vi "释放所有通道.vi"(9 "RF/CLK":string, 11 "TCP Network Connection in":refnum<k5>) -> (0 "error out":errorcluster, 3 "TCP Network Connection out":refnum<k5>)   [LabVIEW 2015]
uses:
  Global/SeverGlobal.vi
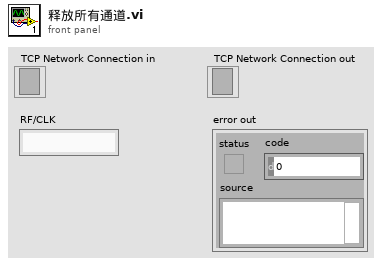
[diagram p1: front panel]
types:
  T1 = typedef "响应消息头.ctl" = string
  T2 = cluster{"TCP Ref":refnum<k5>, "IP":string, "userName":string, "A":u16, "COM":u16, "time":u32}[]
  T3 = cluster{"TCP Ref":refnum<k5>, "Broadcast":refnum<k5>, "TF Ref":refnum<k5>, "IP":string, "port":u16, "userName":string, "passWord":string, "authority":string}[]
  T4 = cluster{"TCP Ref":refnum<k5>, "IP":string, "userName":string, "IN":u16, "OUT":u16, "time":u32}[]
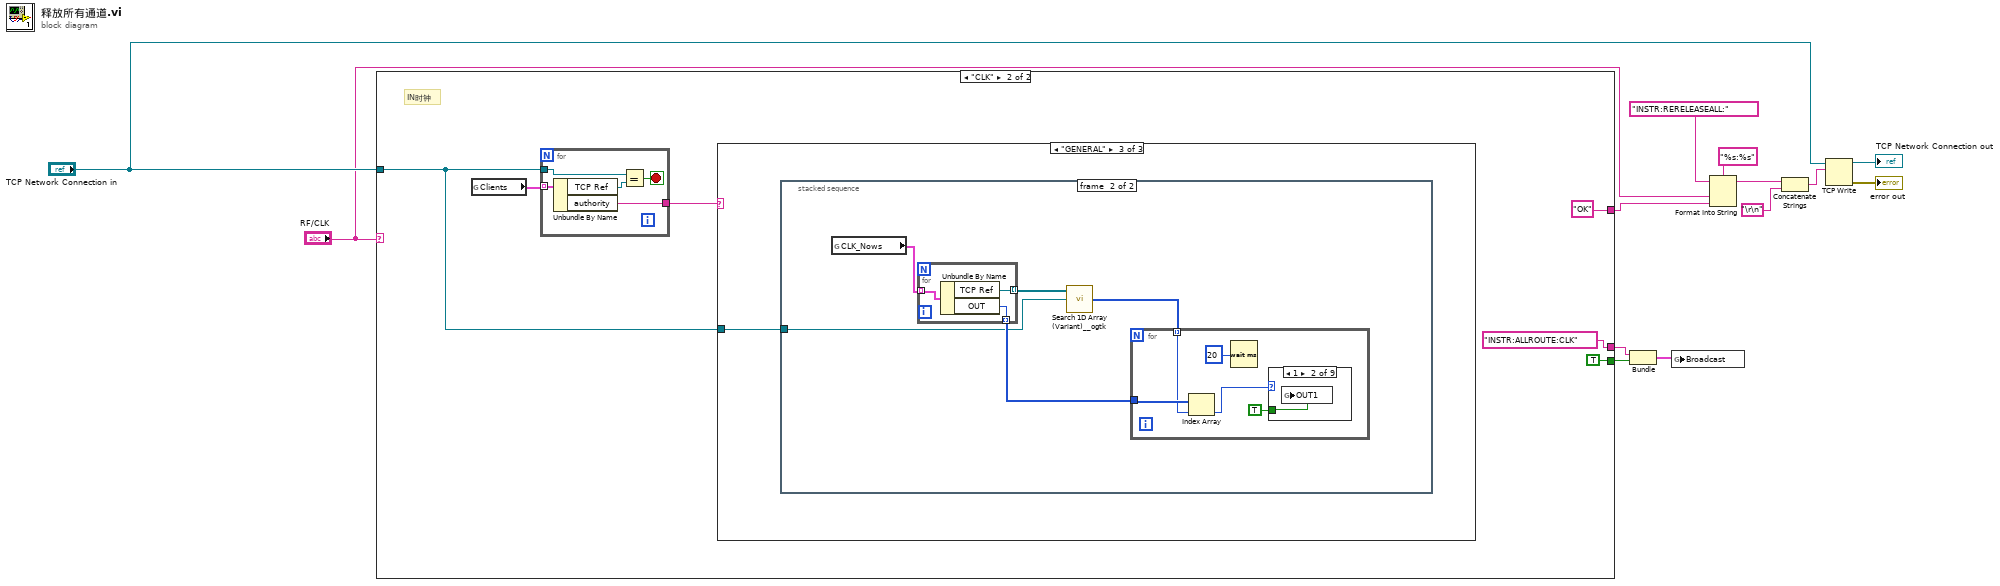
[diagram p0: block diagram]
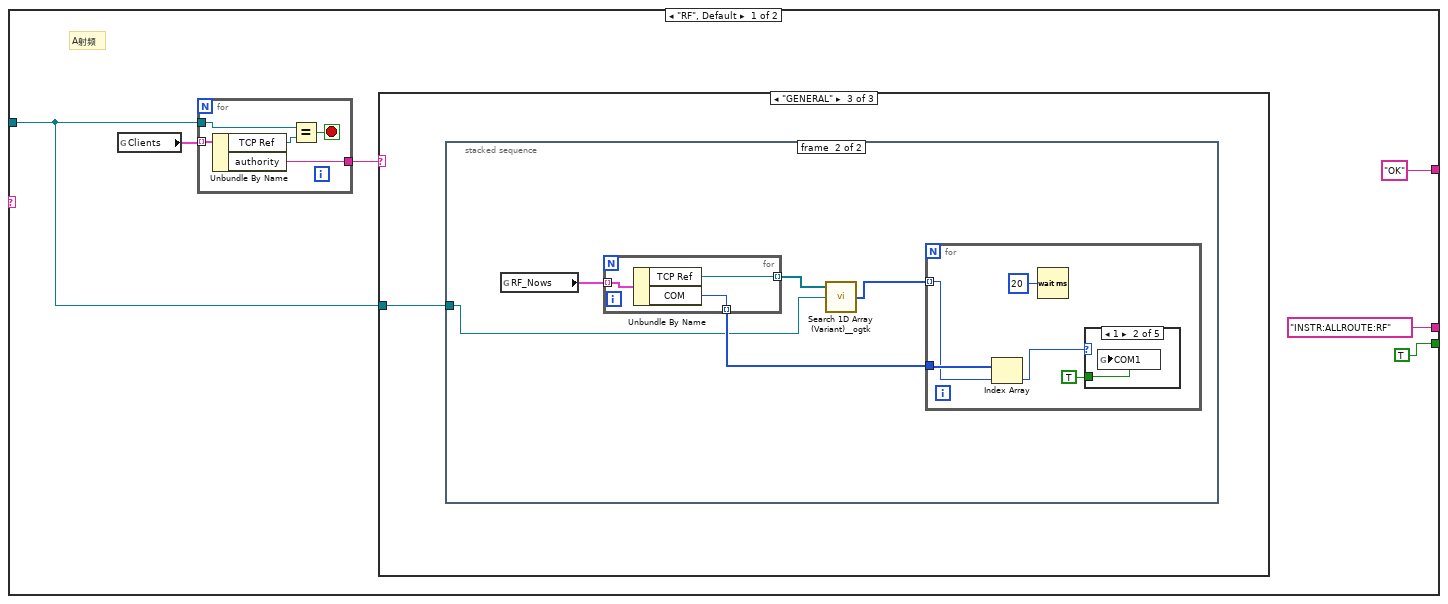
[diagram p2: hidden frame]
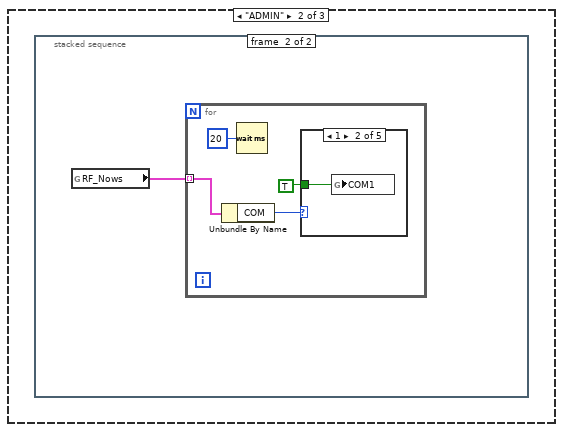
[diagram p4: hidden frame]
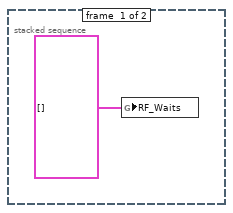
[diagram p5: hidden frame]
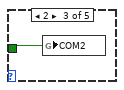
[diagram p7: hidden frame]
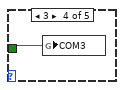
[diagram p8: hidden frame]
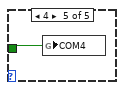
[diagram p9: hidden frame]
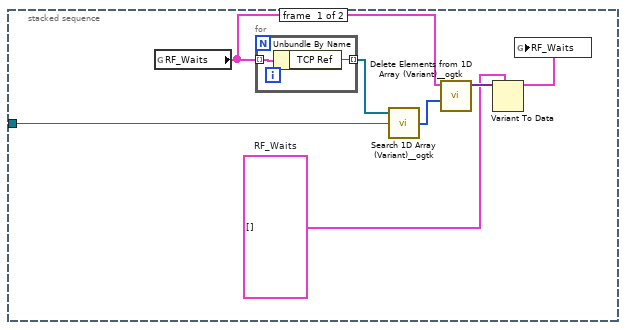
[diagram p10: hidden frame]
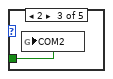
[diagram p12: hidden frame]
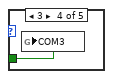
[diagram p13: hidden frame]
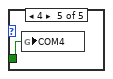
[diagram p14: hidden frame]
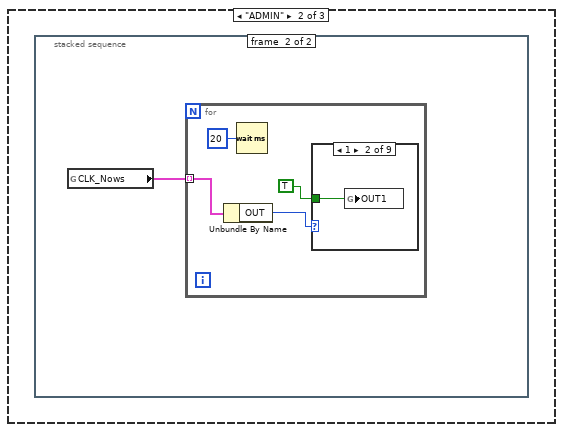
[diagram p16: hidden frame]
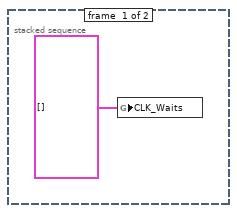
[diagram p17: hidden frame]
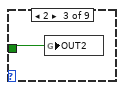
[diagram p19: hidden frame]
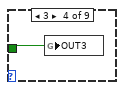
[diagram p20: hidden frame]
diagram:
  n1 = case shown="\"CLK\"" "RF/CLK" {
    tunnel: ["OK" ("format string") "OK" ("format string")] -> w1
    tunnel: "TCP Network Connection in" -> [w14 w62]
    tunnel: ["INSTR:ALLROUTE:RF" ("format string") "INSTR:ALLROUTE:CLK" ("format string")] -> w4
    tunnel: [TRUE TRUE] -> w3
    frame "RF", Default {
      # "A射频"
      n2 = global read "SeverGlobal.vi" "Clients"() -> (w19:T3)
      n3 = for {
        tunnel: w19 -> [w61] mode=indexing
        tunnel: w14 -> [w59]
        tunnel: [w57] -> w18
        stop <- w58 stop-if-true
        n4 = Unbundle By Name(w61) -> ("TCP Ref"=w60:refnum<k5>, "authority"=w57:string)
        n5 = Equal?(x=w59, y=w60) -> (x = y?=w58:bool)
      }
      n6 = case shown="\"GENERAL\"" w18 {
        tunnel: w14 -> [_ _ w30]
        frame "False", Default {
        }
        frame "ADMIN" {
          n7 = stacked-sequence {
            frame #0 {
              n8 = global write "SeverGlobal.vi" "RF_Waits"(T2 [] ("RF_Waits")) -> ()
            }
            frame #1 {
              n9 = global read "SeverGlobal.vi" "RF_Nows"() -> (w21:T2)
              n10 = for {
                tunnel: w21 -> [w25] mode=indexing
                n11 = Unbundle By Name(w25) -> ("COM"=w23:u16)
                n12 = Wait (ms)(milliseconds to wait=u32 20) -> ()  [unwired: 1 out]
                n13 = case shown="1" w23 {
                  tunnel: TRUE ("COM1") -> [_ w26 w27 w28 w29]
                  frame 0, Default {
                  }
                  frame 1 {
                    n14 = global write "SeverGlobal.vi" "COM1"(w26) -> ()
                  }
                  frame 2 {
                    n15 = global write "SeverGlobal.vi" "COM2"(w27) -> ()
                  }
                  frame 3 {
                    n16 = global write "SeverGlobal.vi" "COM3"(w28) -> ()
                  }
                  frame 4 {
                    n17 = global write "SeverGlobal.vi" "COM4"(w29) -> ()
                  }
                }
              }
            }
          }
        }
        frame "GENERAL" {
          n18 = stacked-sequence {
            tunnel: w30 -> [w36 w40]
            frame #0 {
              w32 = T2 []  # RF_Waits
              n19 = global read "SeverGlobal.vi" "RF_Waits"() -> (w34:T2)
              n20 = for {
                tunnel: w34 -> [w39] mode=indexing
                tunnel: [w38] -> w37 mode=indexing
                n21 = Unbundle By Name(w39) -> ("TCP Ref"=w38:refnum<k5>)
              }
              n22 = call <userlib>:"Search 1D Array (Variant)__ogtk.vi"("Array"=w37, "Element Data"=w36) -> ("Indices of Elements"=w35:i32[])  [unwired: 7 in]
              n23 = call <userlib>:"Delete Elements from 1D Array (Variant)__ogtk.vi"("indices"=w35, "array"=w34) -> ("array w/ subset deleted"=w33:variant[])  [unwired: 8 in, 1 out]
              n24 = Variant To Data(type=w32, Variant=w33) -> (data=w31:T2)  [unwired: 1 in, 1 out]
              n25 = global write "SeverGlobal.vi" "RF_Waits"(w31) -> ()
            }
            frame #1 {
              n26 = global read "SeverGlobal.vi" "RF_Nows"() -> (w41:T2)
              n27 = for {
                tunnel: w41 -> [w56] mode=indexing
                tunnel: [w55] -> w42 mode=indexing
                tunnel: [w54] -> w43 mode=indexing
                n28 = Unbundle By Name(w56) -> ("TCP Ref"=w55:refnum<k5>, "COM"=w54:u16)
              }
              n29 = call <userlib>:"Search 1D Array (Variant)__ogtk.vi"("Array"=w42, "Element Data"=w40) -> ("Indices of Elements"=w44:i32[])  [unwired: 7 in]
              n30 = for {
                tunnel: w43 -> [w48]
                tunnel: w44 -> [w47] mode=indexing
                n31 = Index Array(array=w48, index=w47) -> (element=w46:u16)
                n32 = Wait (ms)(milliseconds to wait=u32 20) -> ()  [unwired: 1 out]
                n33 = case shown="1" w46 {
                  tunnel: TRUE -> [_ w50 w51 w52 w53]
                  frame 0, Default {
                  }
                  frame 1 {
                    n34 = global write "SeverGlobal.vi" "COM1"(w50) -> ()
                  }
                  frame 2 {
                    n35 = global write "SeverGlobal.vi" "COM2"(w51) -> ()
                  }
                  frame 3 {
                    n36 = global write "SeverGlobal.vi" "COM3"(w52) -> ()
                  }
                  frame 4 {
                    n37 = global write "SeverGlobal.vi" "COM4"(w53) -> ()
                  }
                }
              }
            }
          }
        }
      }
    }
    frame "CLK" {
      # "IN时钟"
      n38 = global read "SeverGlobal.vi" "Clients"() -> (w67:T3)
      n39 = for {
        tunnel: w67 -> [w117] mode=indexing
        tunnel: w62 -> [w115]
        tunnel: [w113] -> w66
        stop <- w114 stop-if-true
        n40 = Unbundle By Name(w117) -> ("TCP Ref"=w116:refnum<k5>, "authority"=w113:string)
        n41 = Equal?(x=w115, y=w116) -> (x = y?=w114:bool)
      }
      n42 = case shown="\"GENERAL\"" w66 {
        tunnel: w62 -> [_ _ w82]
        frame "False", Default {
        }
        frame "ADMIN" {
          n43 = stacked-sequence {
            frame #0 {
              n44 = global write "SeverGlobal.vi" "CLK_Waits"(T2 [] ("RF_Waits")) -> ()
            }
            frame #1 {
              n45 = global read "SeverGlobal.vi" "CLK_Nows"() -> (w69:T4)
              n46 = for {
                tunnel: w69 -> [w73] mode=indexing
                n47 = Unbundle By Name(w73) -> ("OUT"=w70:u16)
                n48 = Wait (ms)(milliseconds to wait=u32 20) -> ()  [unwired: 1 out]
                n49 = case shown="1" w70 {
                  tunnel: TRUE ("COM1") -> [_ w74 w75 w76 w77 w78 w79 w80 w81]
                  frame 0, Default {
                  }
                  frame 1 {
                    n50 = global write "SeverGlobal.vi" "OUT1"(w74) -> ()
                  }
                  frame 2 {
                    n51 = global write "SeverGlobal.vi" "OUT2"(w75) -> ()
                  }
                  frame 3 {
                    n52 = global write "SeverGlobal.vi" "OUT3"(w76) -> ()
                  }
                  frame 4 {
                    n53 = global write "SeverGlobal.vi" "OUT4"(w77) -> ()
                  }
                  frame 5 {
                    n54 = global write "SeverGlobal.vi" "OUT5"(w78) -> ()
                  }
                  frame 6 {
                    n55 = global write "SeverGlobal.vi" "OUT6"(w79) -> ()
                  }
                  frame 7 {
                    n56 = global write "SeverGlobal.vi" "OUT7"(w80) -> ()
                  }
                  frame 8 {
                    n57 = global write "SeverGlobal.vi" "OUT8"(w81) -> ()
                  }
                }
              }
            }
          }
        }
        frame "GENERAL" {
          n58 = stacked-sequence {
            tunnel: w82 -> [w83 w92]
            frame #0 {
              w88 = T2 []  # CLK_Waits
              n59 = global read "SeverGlobal.vi" "CLK_Waits"() -> (w86:T4)
              n60 = for {
                tunnel: w86 -> [w91] mode=indexing
                tunnel: [w90] -> w84 mode=indexing
                n61 = Unbundle By Name(w91) -> ("TCP Ref"=w90:refnum<k5>)
              }
              n62 = call <userlib>:"Search 1D Array (Variant)__ogtk.vi"("Array"=w84, "Element Data"=w83) -> ("Indices of Elements"=w85:i32[])  [unwired: 7 in]
              n63 = call <userlib>:"Delete Elements from 1D Array (Variant)__ogtk.vi"("indices"=w85, "array"=w86) -> ("array w/ subset deleted"=w87:variant[])  [unwired: 8 in, 1 out]
              n64 = Variant To Data(type=w88, Variant=w87) -> (data=w89:T2)  [unwired: 1 in, 1 out]
              n65 = global write "SeverGlobal.vi" "CLK_Waits"(w89) -> ()
            }
            frame #1 {
              n66 = global read "SeverGlobal.vi" "CLK_Nows"() -> (w94:T4)
              n67 = for {
                tunnel: w94 -> [w112] mode=indexing
                tunnel: [w111] -> w93 mode=indexing
                tunnel: [w110] -> w96 mode=indexing
                n68 = Unbundle By Name(w112) -> ("TCP Ref"=w111:refnum<k5>, "OUT"=w110:u16)
              }
              n69 = call <userlib>:"Search 1D Array (Variant)__ogtk.vi"("Array"=w93, "Element Data"=w92) -> ("Indices of Elements"=w95:i32[])  [unwired: 7 in]
              n70 = for {
                tunnel: w96 -> [w100]
                tunnel: w95 -> [w99] mode=indexing
                n71 = Index Array(array=w100, index=w99) -> (element=w98:u16)
                n72 = Wait (ms)(milliseconds to wait=u32 20) -> ()  [unwired: 1 out]
                n73 = case shown="1" w98 {
                  tunnel: TRUE -> [_ w102 w103 w104 w105 w106 w107 w108 w109]
                  frame 0, Default {
                  }
                  frame 1 {
                    n74 = global write "SeverGlobal.vi" "OUT1"(w102) -> ()
                  }
                  frame 2 {
                    n75 = global write "SeverGlobal.vi" "OUT2"(w103) -> ()
                  }
                  frame 3 {
                    n76 = global write "SeverGlobal.vi" "OUT3"(w104) -> ()
                  }
                  frame 4 {
                    n77 = global write "SeverGlobal.vi" "OUT4"(w105) -> ()
                  }
                  frame 5 {
                    n78 = global write "SeverGlobal.vi" "OUT5"(w106) -> ()
                  }
                  frame 6 {
                    n79 = global write "SeverGlobal.vi" "OUT6"(w107) -> ()
                  }
                  frame 7 {
                    n80 = global write "SeverGlobal.vi" "OUT7"(w108) -> ()
                  }
                  frame 8 {
                    n81 = global write "SeverGlobal.vi" "OUT8"(w109) -> ()
                  }
                }
              }
            }
          }
        }
      }
    }
  }
  n82 = Bundle("format string"=w4, w3) -> (w5:cluster{"format string":string, bool})  [unwired: 1 in]
  n83 = global write "SeverGlobal.vi" "Broadcast"(w5) -> ()
  n84 = Format Into String(format string="%s:%s", initial string=T1 "INSTR:RERELEASEALL:" ("Combo Box"), "RF/CLK", w1) -> (resulting string=w13:string)  [unwired: 1 in, 1 out]
  n85 = Concatenate Strings(w13, "\r\n") -> (w9:string)
  n86 = TCP Write(connection ID="TCP Network Connection in", data in=w9) -> (connection ID out=→"TCP Network Connection out":refnum<k5>, error out=→"error out":errorcluster)  [unwired: 2 in, 1 out]
